vi "GetMetadataValue.vi"(8 "error in (no error)":errorcluster, 10 "key":string, 11 "session id in":i32) -> (0 "error out":errorcluster, 1 "MetadataValue":string, 3 "session id out":i32)   [LabVIEW 2017, in "libonnx_wrapper.lvlib"]
doc: "/**\n * @brief Получить значение метаданных по ключу\n * \n * @param sessionId [IN] ID сессии\n * @param key [IN] Ключ метаданных (например, \"producer_name\")\n * @param buffer [OUT] Буфер для строки со значением\n * @param bufferSize [IN] Размер буфера (рекомендуется 256)\n * \n * @return int32: 0 при успехе\n * @return int32: -1 если ключ не найден\n */\nint GetMetadataValue(int sessionId, const char* key, char* buffer, int bufferSize);"
uses:
  libonnx_wrapper.lvlib
panel:
  out "bufferSize":i32
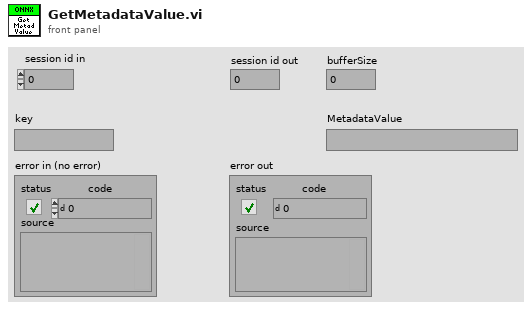
[diagram p1: front panel]
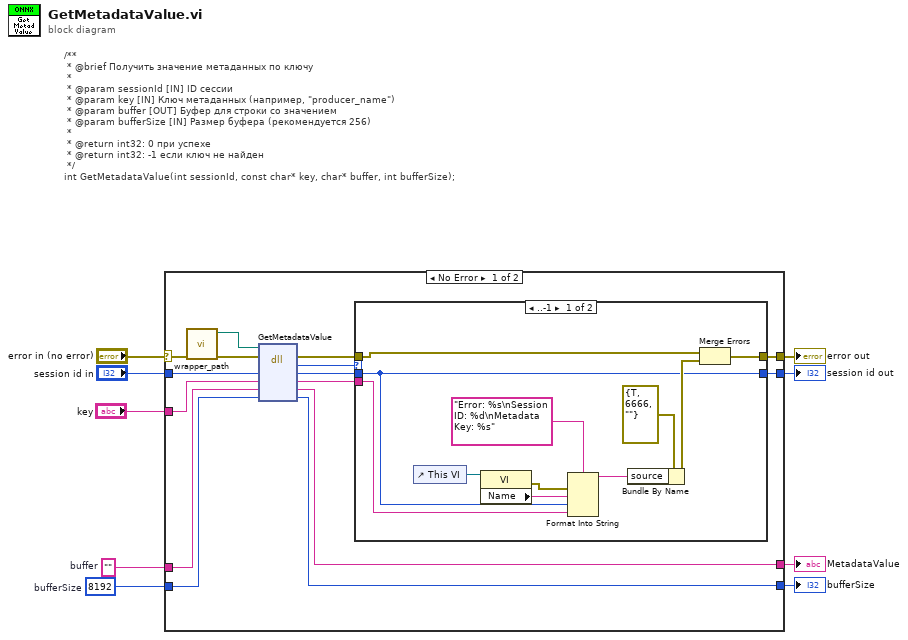
[diagram p0: block diagram]
diagram:
  w6 = 8192  # bufferSize
  w7 = ""  # buffer
  # "/**\n * @brief Получить значение метаданных по ключу\n * \n * @param sessionId [IN] ID сессии\n * @param key [IN] Ключ метаданных (например, \"producer_name\")\n * @param buffer [OUT] Буфер для строки со значением\n * @param bufferSize [IN] Размер буфера (рекомендуется 256)\n * \n * @return int32: 0 при успехе\n * @return int32: -1 если ключ не найден\n */\nint GetMetadataValue(int sessionId, const char* key, char* buffer, int bufferSize);"
  n1 = case shown="No Error" "error in (no error)" {
    selector: "error in (no error)" -> [w10 w39]
    tunnel: "session id in" -> [w22 w38]
    tunnel: "key" -> [w21 _]
    tunnel: w7 -> [w20 _]
    tunnel: w6 -> [w19 _]
    tunnel: [w18 _] -> w5
    tunnel: [w17 _] -> w4
    tunnel: [w15 w39] -> w3
    tunnel: [w14 w38] -> w2
    frame No Error {
      n2 = call "wrapper_path.vi"("error in (no error)"=w10) -> ("error out"=w24:errorcluster, "wrapper path"=w23:path)  [unwired: 9 in]
      n3 = dll-call lib="home/ivan/LabVIEWData/ONNX/Test/libonnx_wrapper/unix64/libonnx_wrapper.*" fn="GetMetadataValue"(path in=w23, error in=w24, "sessionId"=w22, "key"=w21, "buffer"=w20, "bufferSize"=w19) -> (error out=w16:errorcluster, "return"=w13:i32, "sessionId"=w12:i32, "key"=w11:string, "buffer"=w18:string, "bufferSize"=w17:i32)  [unwired: 1 in, 1 out]
      n4 = case shown="..-1" w13 {
        tunnel: w16 -> [w26 w37]
        tunnel: [w27 w37] -> w15
        tunnel: w12 -> [w28 w36]
        tunnel: [w28 w36] -> w14
        tunnel: w11 -> [w25 _]
        frame ..-1 {
          n5 = control-ref of="This VI"() -> (w32:refnum<vi>)
          n6 = property class="VI"(reference=w32) -> (error out=w29:errorcluster, "Name"=w31:string)  [unwired: 1 in, 1 out]
          n7 = Format Into String(format string="Error: %s\nSession ID: %d\nMetadata Key: %s", error in=w29, w31, w28, w25) -> (resulting string=w33:string)  [unwired: 1 in, 1 out]
          n8 = Bundle By Name(cluster=errorcluster {"status"=TRUE, "code"=6666, "source"=""} ("error out"), "source"=w33) -> (w34:errorcluster)
          n9 = Merge Errors(w26, w34) -> (w27:errorcluster)
        }
        frame 0.. {
        }
      }
    }
    frame Error {
    }
  }
  "error out" <- w3
  "session id out" <- w2
  "MetadataValue" <- w5
  "bufferSize" <- w4
